vi "2 Tap 14-Bit.vi"() -> (0 "PixelData":cluster{"Pixel 0":u16, "Pixel 1":u16})   [LabVIEW 2014]
uses:
  <vilib>/rvi/eio/common/nirviEmuTemplateMethod_errors.vi
  <vilib>/eio/EIONode/EIONode.xnode
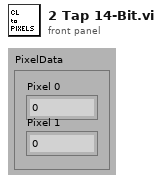
[diagram p1: front panel]
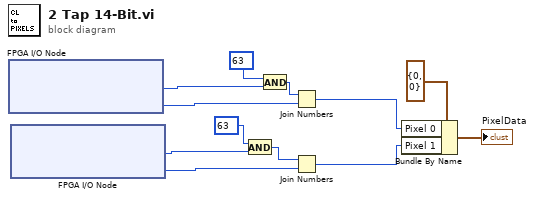
[diagram p0: block diagram]
diagram:
  n1 = xnode "FPGA I/O Node"() -> ("IO Module\\CL Port B"=w6:u8, "IO Module\\CL Port A"=w5:u8)  [unwired: 2 in, 2 out]
  n2 = xnode "FPGA I/O Node"() -> ("IO Module\\CL Port E"=w4:u8, "IO Module\\CL Port D"=w3:u8)  [unwired: 2 in, 2 out]
  n3 = And(x=u8 63 ("hi"), y=w4) -> (x .and. y?=w7:u8)
  n4 = And(x=u8 63 ("hi"), y=w6) -> (x .and. y?=w9:u8)
  n5 = Join Numbers(hi=w9, lo=w5) -> ((hi.lo)=w2:u16)
  n6 = Join Numbers(hi=w7, lo=w3) -> ((hi.lo)=w1:u16)
  n7 = Bundle By Name(cluster=cluster{"Pixel 0":u16, "Pixel 1":u16} {"Pixel 0"=0, "Pixel 1"=0} ("PixelData"), "Pixel 0"=w2, "Pixel 1"=w1) -> (→"PixelData":cluster{"Pixel 0":u16, "Pixel 1":u16})
